vi "Bind To Type - LabVIEW Object - Type Is LabVIEW Object.vi"() -> ()   [LabVIEW 2017, in "Default Serialization Binder Tests.lvlib"]
uses:
  Default Serialization Binder Tests.lvlib
  Default Serialization Binder/Default Serialization Binder.lvclass
  <vilib>/addons/_JKI Toolkits/Caraya/classes/Assert/Assert Equal Value and Type_Variant.vi
  <vilib>/addons/_JKI Toolkits/Caraya/classes/Test/Test.lvclass
  <vilib>/addons/_JKI Toolkits/Caraya/classes/Assert/Assert.lvclass
panel:
  out "error out":errorcluster
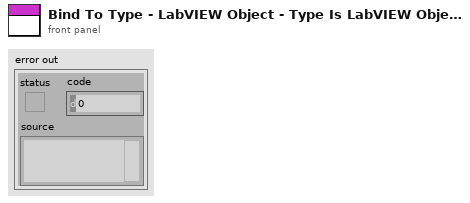
[diagram p1: front panel]
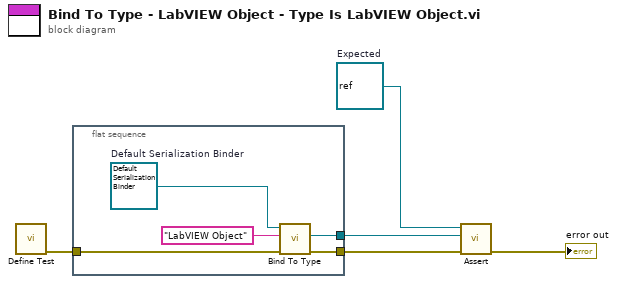
[diagram p0: block diagram]
diagram:
  w1 = refnum<class> refnum  # Expected
  n1 = call <vilib>:"Define Test.vi"() -> ("error out"=w3:errorcluster)  [unwired: 11 in]
  n2 = flat-sequence {
    tunnel: [w8] -> w2
    tunnel: [w6] -> w4
    tunnel: w3 -> [w7]
    frame #0 {
      w10 = refnum<class "Default Serialization Binder.lvclass"> refnum  # Default Serialization Binder
      n3 = call-dynamic "Bind To Type.vi"("error in (no error)"=w7, "Type Name"="LabVIEW Object", "Default Serialization Binder in"=w10) -> ("error out"=w6:errorcluster, "Type"=w8:refnum<class>)  [unwired: 6 in, 1 out]
    }
  }
  n4 = call-poly <vilib>:"Assert.vi"("error in (no error)"=w4, "Y"=w2, "X"=w1) -> ("error out"=→"error out":errorcluster)  [unwired: 8 in]
